vi "Examples ZoomAtClickPosition.vi"() -> ()   [LabVIEW 2020, in "LcPictureBox.lvclass"]
uses:
  LcPictureBox.lvclass
  Pen.ctl
  Font.ctl
  CallBackVIs/CallBAck_MouseDown.vi
  System.Windows.Forms
panel:
  in  "PictureBox":refnum<k24>(container)
  out "MouseMove":cluster{"X":i32, "Y":i32, "Button":i32}
  in  "Origin":cluster{"x":sgl, "y":sgl}
  out "MouseDown":cluster{"X":i32, "Y":i32, "Button":i32}
  in  "Scale":sgl=0.1 min=0.1 max=10 step=0.5
  out "Error Out":errorcluster
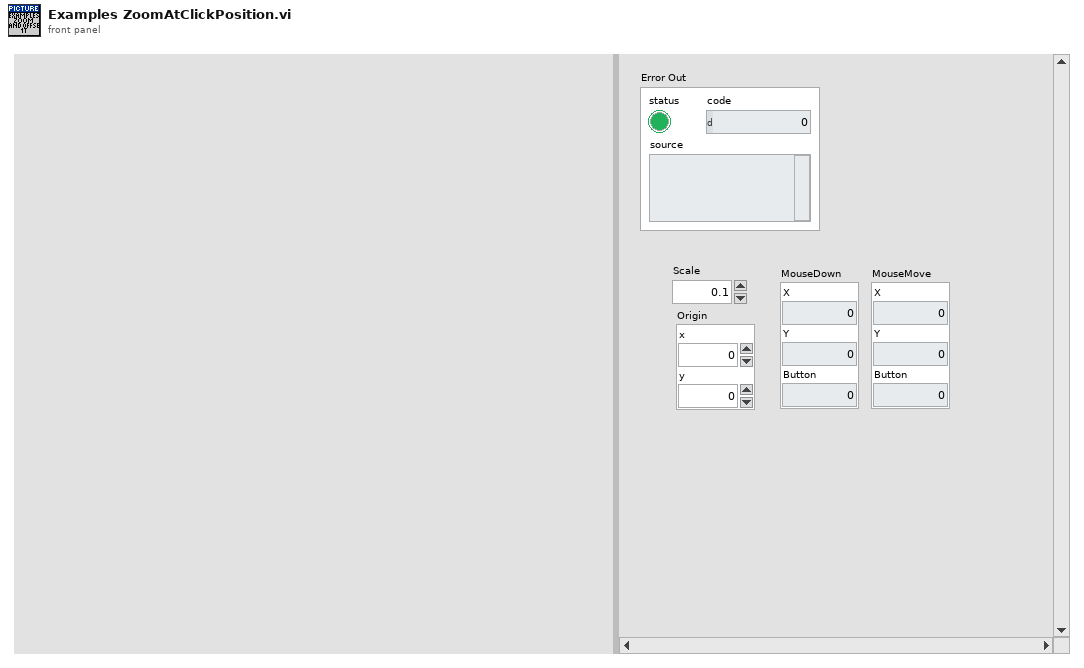
[diagram p1: front panel]
types:
  T1 = typedef "LcPictureBox.lvclass/Pen.ctl" = cluster{"Width":u16, "Style":enum32{"Solid", "Dash", "Dot", "DashDot", "DashDotDot"}}
  T2 = cluster{"horizontal":enum16{"Left", "Center", "Right"}, "vertical":enum16{"Top", "Center", "Bottom"}}
  T3 = typedef "LcPictureBox.lvclass/Font.ctl" = cluster{"FontName":string, "Size(Pts)":dbl, "Style":enum16{"Regular", "Bold", "Italic", "Underline", "Strikeout"}}
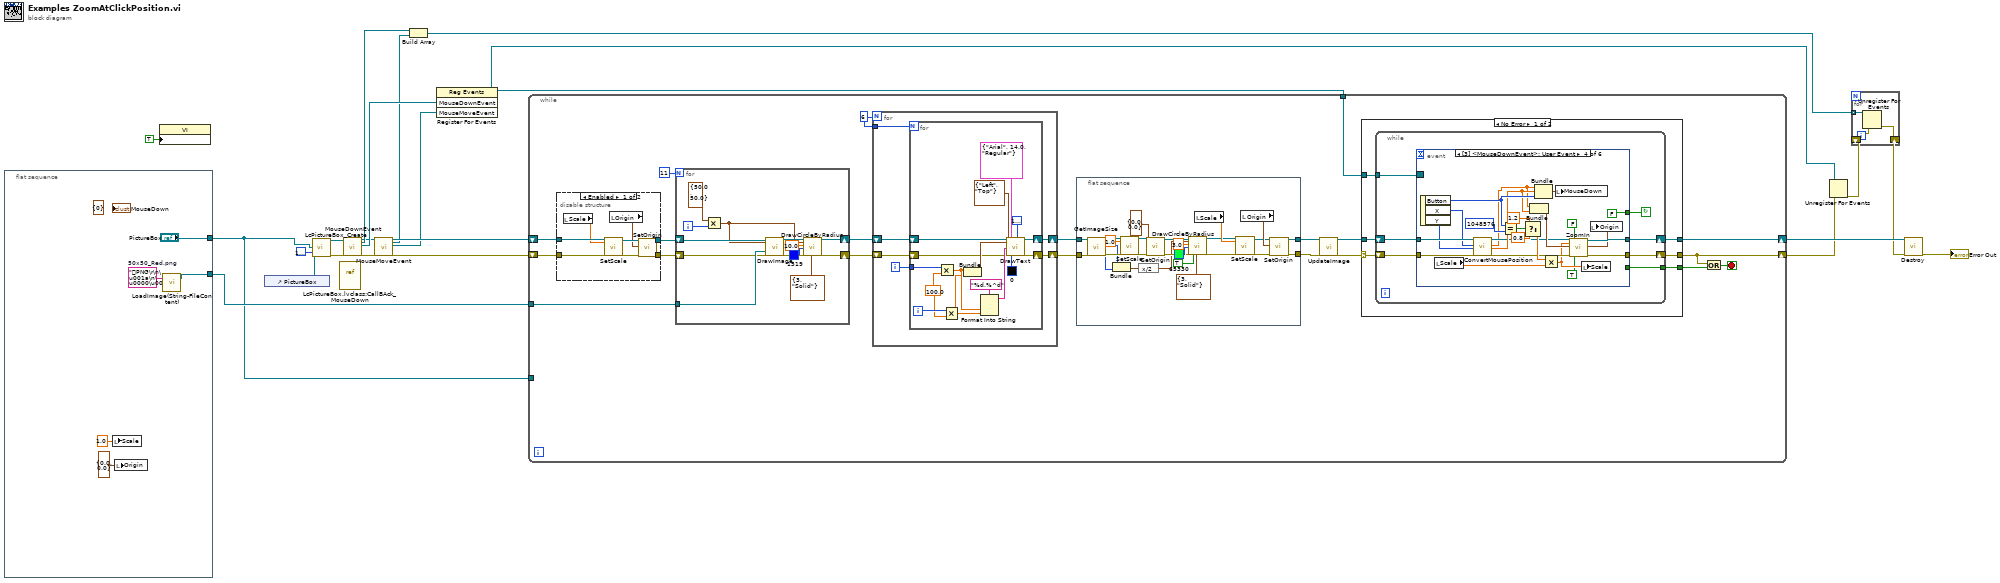
[diagram p0: block diagram]
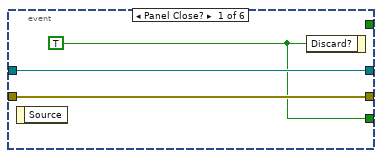
[diagram p3: hidden frame]
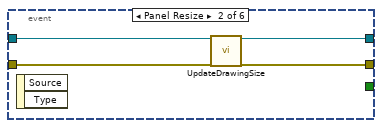
[diagram p4: hidden frame]
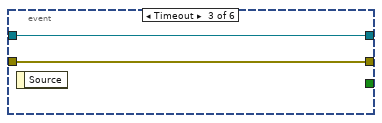
[diagram p5: hidden frame]
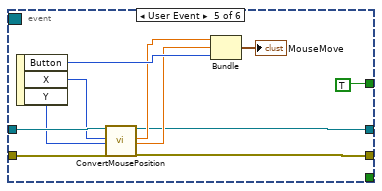
[diagram p6: hidden frame]
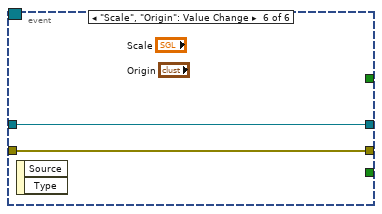
[diagram p7: hidden frame]
diagram:
  n1 = flat-sequence {
    tunnel: [w26] -> w21
    tunnel: ["PictureBox"] -> w1
    frame #0 {
      (unwired) cluster{"Button":i32} {"Button"=0} ("MouseInfo")
      w24 = "PNG\r\n\u001a\n\u0000\u0000\u0000\rIHDR\u0000\u0000\u00002\u0000\u0000\u00002\b\u0006\u0000\u0000\u0000\u001e?±\u0000\u0000\u0000\u0001sRGB\u0000®Î\u001cé\u0000\u0000\u0000\u0004gAMA\u0000\u0000±\u000büa\u0005\u0000\u0000\u0000\tpHYs\u0000\u0000\u000eÄ\u0000\u0000\u000eÄ\u0001+\u000e\u001b\u0000\u0000\u0002IDAThCí1kÛ@\u0018ß\u0016I\bä\u0018Å\u0016M\u0003b\u001a:tþA¡¦ £Wgèbºeö¥C¼zÌÖ©dÈ?ÈÞ¡¤ ­p\"ú°\u0005íw§S­Z\u0004Û­k¸\u0007ÌY§;½zï¾ï;\u001fÝ´ö~â\u0001ðX¶ÿ=Újh#ª¡¨6¢\u001aÚjh#ª¡¨6¢\u001aÚj³§1:_'¸9]o\u000fÇ¶¼ ÆIÃÉ\u001cg£ëîà¸f«µ¨Xçþ\u001d±êè:Ï\u000bCösèáûüá4fàyèZ\tFñ\u0015:Ó¹\u001c°\u0001\u0015éw&7iòòÊ,c\u0018^áhVÇië\t^>~p\u0011}+¨Xgó\u001cI\u0019>Ì¨uÂ\u001c¼qx;ÃeJá0\rÐ\f.Ñ¸ËÉûÖÞµ5tS>\u001b\u0018MèEøË\u0004\u0001úIAîóxõM+»<7ù²&øL\u0002íÚ\u000e\u0006ü60\u0014\fïãÂÈÃï*twÄ¨QBíâbràØðiÒh²iüè5<1÷è;Ãù4¢p°1h¸hË\u0011Õè,(\u0019iÛ.U\u0005ÚNj{Û-=å/\u0004\\ü`\u0018gCÖÃpqâÒê±k\u001cÐnøTmzD®LG²:G\f\u0013/åWaeó,4r¾Ì)thÕÿ¨:ð:«¤s|â­ifa\u000b2\n\u0019Þ\n\u0018>ò¼¶jx\u000bÐ9qÈóÂÙ¥Ð¡\u0017¿É|¹¿ÕG\u0001:QaB\u001f..."  # 50x50_Red.png
      n2 = local write "Scale"(sgl 1.0 ("Scale")) -> ()
      n3 = local write "Origin"(cluster{"x":sgl, "y":sgl} {"x"=0.0, "y"=0.0} ("Origin")) -> ()
      n4 = call "LoadImage(String-FileContent).vi"("ImageFileContent"=w24) -> ("ImageOut"=w26:refnum<k24>)  [unwired: 16 in, 2 out]
    }
  }
  n5 = property class="VI"("Front Panel.IsFrontmost"=TRUE ("Front Panel Window:Is Frontmost")) -> ()  [unwired: 2 in, 2 out]
  n6 = control-ref of="PictureBox"() -> (w17:refnum<vi>)
  n7 = call "LcPictureBox_Create.vi"("PictureBox"=w1, "PictureBoxActiveXReference"=w17, "BgColor(None)"=u32 16777216) -> ("reference out"=w19:refnum<class "LcPictureBox.lvclass">, "Error Out"=w20:errorcluster)  [unwired: 14 in, 1 out]
  n8 = vi-ref "LcPictureBox.lvclass:CallBAck_MouseDown.vi"() -> ()  [unwired: 1 out]
  n9 = call-dynamic "MouseDownEvent.vi"("reference in"=w19, "error in (no error)"=w20) -> ("reference out"=w6:refnum<class "LcPictureBox.lvclass">, "Event Callback Refnum"=w11:refnum<k27>, "MouseDownEvent"=w18:refnum<user-event>, "error out"=w12:errorcluster)  [unwired: 14 in]
  n10 = call-dynamic "MouseMoveEvent.vi"("reference in"=w6, "error in (no error)"=w12) -> ("reference out"=w5:refnum<class "LcPictureBox.lvclass">, "Event Callback Refnum"=w2:refnum<k27>, "MouseMoveEvent"=w4:refnum<user-event>, "error out"=w7:errorcluster)  [unwired: 14 in]
  n11 = Build Array(w11, w2) -> (w3:refnum<k27>[])
  n12 = register-events(w18, w4) -> (reference out=w15:refnum<event-registration>)  [unwired: 2 in, 1 out]
  n13 = while {
    tunnel: w21 -> [w46]
    tunnel: w15 -> [w44]
    shift-right: [w43] -> w14
    shift-left: w5 -> [w45]
    shift-right: [w40] -> w10
    shift-left: w7 -> [w41]
    tunnel: w1 -> [_]
    stop <- w38 stop-if-true
    w34 = 6
    n14 = disable-structure shown="Enabled" {
      disable-tunnel: w45 -> [w80 w81]
      disable-tunnel: w41 -> [w79 w82]
      disable-tunnel: [w76 w82] -> w37
      disable-tunnel: [w75 w81] -> w36
      frame Enabled {
        n15 = local read "Scale"() -> (w74:sgl)
        n16 = call-dynamic "SetScale.vi"("reference in"=w80, "ScaleFactor"=w74, "Error In"=w79) -> ("reference out"=w78:refnum<class "LcPictureBox.lvclass">, "Error Out"=w77:errorcluster)  [unwired: 15 in]
        n17 = local read "Origin"() -> (w73:cluster{"x":sgl, "y":sgl})
        n18 = call-dynamic "SetOrigin.vi"("reference in"=w78, "Origin"=w73, "Error In"=w77) -> ("reference out"=w75:refnum<class "LcPictureBox.lvclass">, "Error Out"=w76:errorcluster)  [unwired: 15 in]
      }
      frame Disabled {
      }
    }
    n19 = for {
      N: 11 -> [_]
      tunnel: w46 -> [w95]
      shift-right: [w87] -> w33
      shift-left: w36 -> [w93]
      shift-right: [w89] -> w32
      shift-left: w37 -> [w94]
      i -> [w92]
      n20 = Multiply(x=cluster{"x":sgl, "y":sgl} {"x"=50.0, "y"=50.0} ("UpperLeftCorner"), y=w92) -> (x*y=w86:cluster{"x":sgl, "y":sgl})
      n21 = call-dynamic "DrawImage.vi"("reference in"=w93, "UpperLeftCorner(0,0)"=w86, "Image"=w95, "Error In"=w94) -> ("reference out"=w88:refnum<class "LcPictureBox.lvclass">, "Error Out"=w90:errorcluster)  [unwired: 14 in]
      n22 = call-dynamic "DrawCircleByRadius.vi"("reference in"=w88, "Center"=w86, "Radius"=sgl 10.0, "Color(Black)"=u32 1519, "Error In"=w90, "Pen(Width=1, Solid)"=T1 {"Width"=3, "Style"=enum."Solid"}) -> ("reference out"=w87:refnum<class "LcPictureBox.lvclass">, "Error Out"=w89:errorcluster)  [unwired: 12 in]
    }
    n23 = for {
      N: w34 -> [_]
      tunnel: w34 -> [w98]
      shift-right: [w100] -> w27
      shift-left: w32 -> [w96]
      shift-right: [w101] -> w28
      shift-left: w33 -> [w97]
      i -> [w99]
      n24 = for {
        N: w98 -> [_]
        tunnel: w99 -> [w111]
        shift-right: [w116] -> w100
        shift-left: w96 -> [w102]
        shift-right: [w117] -> w101
        shift-left: w97 -> [w103]
        i -> [w110]
        w109 = sgl 100.0 ("Y")
        n25 = Multiply(x=w111, y=w109) -> (x*y=w108:sgl)
        n26 = Multiply(x=w110, y=w109) -> (x*y=w107:sgl)
        n27 = Bundle(w108, w107) -> (w104:cluster{sgl, sgl})  [unwired: 1 in]
        n28 = Format Into String(format string="%d,%^d", w108, w107) -> (resulting string=w105:string)  [unwired: 2 in, 1 out]
        n29 = call-dynamic "DrawText.vi"("reference in"=w103, "Origin"=w104, "Alignment(Left,Top)"=T2 {"horizontal"=enum."Left", "vertical"=enum."Top"}, "Text"=w105, "Error In"=w102, "Font(Arial,14pts,Regular)"=T3 {"FontName"="Arial", "Size(Pts)"=14.0, "Style"=enum."Regular"}, "Color(Black)"=u32 0 ("BgColor(Transparent)"), "BgColor(Transparent)"=u32 16777216) -> ("reference out"=w117:refnum<class "LcPictureBox.lvclass">, "Error Out"=w116:errorcluster)  [unwired: 10 in]
      }
    }
    n30 = flat-sequence {
      tunnel: [w68] -> w30
      tunnel: [w67] -> w29
      tunnel: w28 -> [w66]
      tunnel: w27 -> [w65]
      frame #0 {
        n31 = call-dynamic "GetImageSize.vi"("reference in"=w66, "error in (no error)"=w65) -> ("reference out"=w60:refnum<class "LcPictureBox.lvclass">, "Width"=w52:i32, "Height"=w51:i32, "error out"=w59:errorcluster)  [unwired: 14 in]
        n32 = Bundle("Width"=w52, "Height"=w51) -> (w50:cluster{"Width":i32, "Height":i32})  [unwired: 1 in]
        n33 = call-dynamic "SetScale.vi"("reference in"=w60, "ScaleFactor"=sgl 1.0, "Error In"=w59) -> ("reference out"=w58:refnum<class "LcPictureBox.lvclass">, "Error Out"=w61:errorcluster)  [unwired: 15 in]
        n34 = expression code="x/2"(w50) -> (w49:cluster{"Width":i32, "Height":i32})
        n35 = call-dynamic "SetOrigin.vi"("reference in"=w58, "Origin"=cluster{"x":sgl, "y":sgl} {"x"=0.0, "y"=0.0}, "Error In"=w61) -> ("reference out"=w55:refnum<class "LcPictureBox.lvclass">, "Error Out"=w54:errorcluster)  [unwired: 15 in]
        n36 = call-dynamic "DrawCircleByRadius.vi"("reference in"=w55, "Center"=w49, "Radius"=sgl 3.0, "Color(Black)"=u32 65330, "Error In"=w54, "Fill(False)"=TRUE, "Pen(Width=1, Solid)"=T1 {"Width"=3, "Style"=enum."Solid"}) -> ("reference out"=w48:refnum<class "LcPictureBox.lvclass">, "Error Out"=w47:errorcluster)  [unwired: 11 in]
        n37 = local read "Scale"() -> (w71:sgl)
        n38 = call-dynamic "SetScale.vi"("reference in"=w48, "ScaleFactor"=w71, "Error In"=w47) -> ("reference out"=w69:refnum<class "LcPictureBox.lvclass">, "Error Out"=w70:errorcluster)  [unwired: 15 in]
        n39 = local read "Origin"() -> (w72:cluster{"x":sgl, "y":sgl})
        n40 = call-dynamic "SetOrigin.vi"("reference in"=w69, "Origin"=w72, "Error In"=w70) -> ("reference out"=w68:refnum<class "LcPictureBox.lvclass">, "Error Out"=w67:errorcluster)  [unwired: 15 in]
      }
    }
    n41 = call-dynamic "UpdateImage.vi"("reference in"=w30, "Error In"=w29) -> ("reference out"=w42:refnum<class "LcPictureBox.lvclass">, "Error Out"=w31:errorcluster)  [unwired: 14 in, 2 out]
    n42 = case shown="No Error" w31 {
      selector: w31 -> [w123 w178]
      tunnel: w42 -> [w122 w177]
      tunnel: w44 -> [w121 _]
      tunnel: [w120 w178] -> w40
      tunnel: [w119 w177] -> w43
      tunnel: [w118 _] -> w39
      frame No Error {
        n43 = while {
          tunnel: w121 -> [w128]
          shift-right: [w127] -> w120
          shift-left: w123 -> [w130]
          shift-right: [w126] -> w119
          shift-left: w122 -> [w129]
          tunnel: [w124] -> w118
          stop <- w125 continue-if-true
          n44 = event shown="[3] <MouseDownEvent>: User Event" {
            selector: w128 -> [_ _ _ _ _ _]
            dyn-events: _ -> [_ _ _ _ _ _]
            timeout: _ -> [_ _ _ _ _ _]
            tunnel: w130 -> [w133 w137 w138 w148 w170 w175]
            tunnel: [w133 w136 w138 w159 w166 w175] -> w127
            tunnel: w129 -> [w132 w135 w139 w151 w172 w176]
            tunnel: [w132 w134 w139 w160 w165 w176] -> w126
            tunnel: [_ _ _ FALSE TRUE _] -> w125
            tunnel: [w131 _ _ _ _ _] -> w124
            event Panel Close? {
              w131 = TRUE ("Discard?")
              n45 = event-data() -> ()  [unwired: 1 in, 1 out]
              n46 = event-data("Discard?"=w131) -> ()  [unwired: 1 in, 1 out]
            }
            event Panel Resize {
              n47 = event-data() -> ()  [unwired: 1 in, 2 out]
              n48 = call-dynamic "UpdateDrawingSize.vi"("reference in"=w135, "Error In"=w137) -> ("reference out"=w134:refnum<class "LcPictureBox.lvclass">, "Error Out"=w136:errorcluster)  [unwired: 16 in]
            }
            event Timeout {
              n49 = event-data() -> ()  [unwired: 1 in, 1 out]
            }
            event User Event {
              n50 = event-data() -> ("Button"=w162:i32, "X"=w146:i32, "Y"=w145:i32)  [unwired: 1 in]
              n51 = local read "Scale"() -> (w144:sgl)
              n52 = call-dynamic "ConvertMousePosition.vi"("reference in"=w151, "X"=w146, "Y"=w145, "Error In"=w148) -> ("reference out"=w147:refnum<class "LcPictureBox.lvclass">, "X-Out"=w141:sgl, "Y-Out"=w150:sgl, "Error Out"=w149:errorcluster)  [unwired: 12 in]
              n53 = Equal?(x=w162, y=1048576) -> (x = y?=w156:bool)
              n54 = Select(t=1.2, s=w156, f=0.8) -> (s? t:f=w153:dbl)
              n55 = Bundle("X-Out"=w141, "Y-Out"=w150) -> (w157:cluster{"X-Out":sgl, "Y-Out":sgl})  [unwired: 1 in]
              n56 = Bundle("X-Out"=w141, "Y-Out"=w150, "Button"=w162) -> (w158:cluster{"X-Out":sgl, "Y-Out":sgl, "Button":i32})  [unwired: 1 in]
              n57 = Multiply(x=w153, y=w144) -> (x*y=w143:dbl)
              n58 = local write "MouseDown"(w158) -> ()
              n59 = call-dynamic "ZoomIn.vi"("reference in"=w147, "NewScaleValue"=w143, "MousePosition(scaled)"=w157, "Error In"=w149, "ZoomAtMouse"=FALSE, "OnlyCaluclateNewValues"=TRUE) -> ("reference out"=w160:refnum<class "LcPictureBox.lvclass">, "Origin"=w152:cluster{"x":sgl, "y":sgl}, "Error Out"=w159:errorcluster)  [unwired: 10 in, 1 out]
              n60 = local write "Scale"(w143) -> ()
              n61 = local write "Origin"(w152) -> ()
            }
            event User Event {
              n62 = event-data() -> ("Button"=w173:i32, "X"=w168:i32, "Y"=w167:i32)  [unwired: 1 in]
              n63 = call-dynamic "ConvertMousePosition.vi"("reference in"=w172, "X"=w168, "Y"=w167, "Error In"=w170) -> ("reference out"=w165:refnum<class "LcPictureBox.lvclass">, "X-Out"=w169:sgl, "Y-Out"=w171:sgl, "Error Out"=w166:errorcluster)  [unwired: 12 in]
              n64 = Bundle("X-Out"=w169, "Y-Out"=w171, "Button"=w173) -> (→"MouseMove":cluster{"X-Out":sgl, "Y-Out":sgl, "Button":i32})  [unwired: 1 in]
            }
            event "Scale", "Origin": Value Change {
              n65 = event-data() -> ()  [unwired: 1 in, 2 out]
            }
          }
        }
      }
      frame Error {
      }
    }
    n66 = Or(x=w40, y=w39) -> (x .or. y?=w38:bool)
  }
  n67 = Unregister For Events(event registration refnum=w15, error in=w10) -> (error out=w8:errorcluster)
  n68 = for {
    tunnel: w3 -> [w179] mode=indexing
    shift-right: [w181] -> w9
    shift-left: w8 -> [w180]
    n69 = Unregister For Events(event registration refnum=w179, error in=w180) -> (error out=w181:errorcluster)
  }
  "Error Out" <- w9
  n70 = call-dynamic "Destroy.vi"("reference in"=w14, "Error In"=w9) -> ()  [unwired: 16 in, 2 out]
